vi "getPIDGains.vi"(8 "error in (no error)":errorcluster, 11 "PressureServoActuatorClosed in":refnum<class "PressureServoActuatorClosed.lvclass">) -> (0 "error out":errorcluster, 2 "PID gains":T1={"proportional gain (Kc)"=1.0, "integral time (Ti, min)"=0.01, "derivative time (Td, min)"=0.0}, 3 "PressureServoActuatorClosed out":refnum<class "PressureServoActuatorClosed.lvclass">)   [LabVIEW 2015, in "PressureServoActuatorClosed.lvclass"]
uses:
  PressureServoActuatorClosed.lvclass
  PressureServoActuatorClosed.lvclass/PressureServoActuatorClosed.ctl
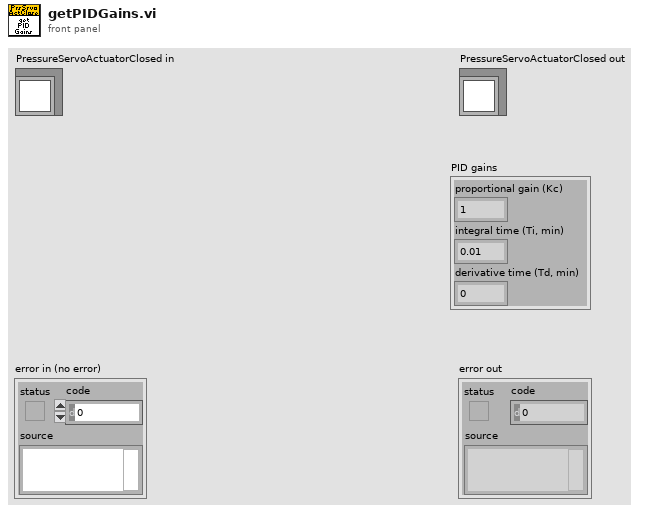
[diagram p1: front panel]
types:
  T1 = cluster{"proportional gain (Kc)":dbl, "integral time (Ti, min)":dbl, "derivative time (Td, min)":dbl}
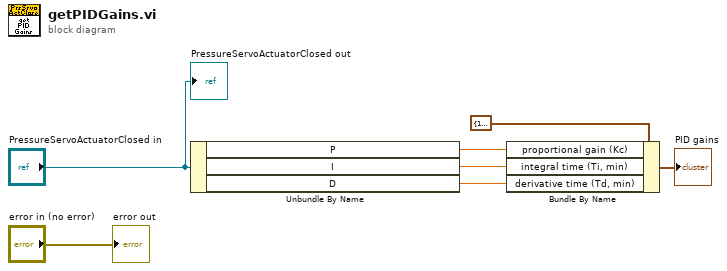
[diagram p0: block diagram]
diagram:
  n1 = Unbundle By Name("PressureServoActuatorClosed in") -> ("P"=w3:dbl, "I"=w2:dbl, "D"=w1:dbl)
  n2 = Bundle By Name(cluster=T1 {"proportional gain (Kc)"=1.0, "integral time (Ti, min)"=0.01, "derivative time (Td, min)"=0.0} ("PID gains"), "proportional gain (Kc)"=w3, "integral time (Ti, min)"=w2, "derivative time (Td, min)"=w1) -> (→"PID gains":T1)
  "error out" <- "error in (no error)"
  "PressureServoActuatorClosed out" <- "PressureServoActuatorClosed in"
